vi "autoToteGrab.vi"(8 "potValue":dbl, 9 "# of totes mode":dbl, 10 "ultrasonic":dbl, 11 "Target tracking data":T1) -> (0 "liftMotorOut":dbl, 1 "holonomicRot":dbl, 2 "holonomicY":dbl, 3 "holonomicX":dbl)   [LabVIEW 2014]
uses:
  Robot Global Data.vi
panel:
  in  "totesGrabbed":dbl
  in  "time":dbl
  in  "State":T2(ring)
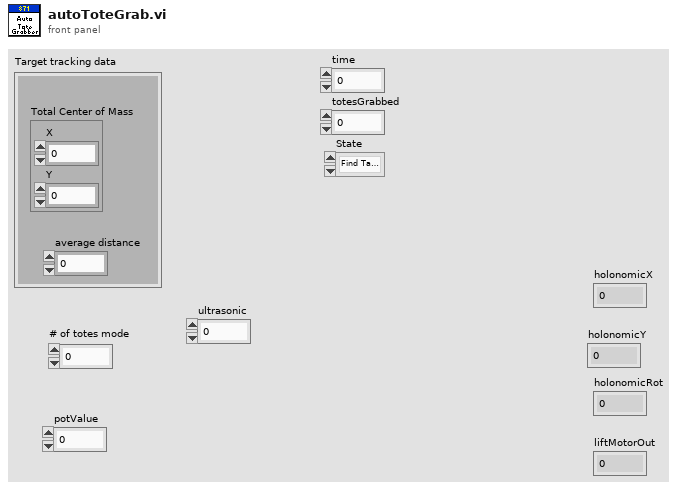
[diagram p1: front panel]
types:
  T1 = cluster{"Total Center of Mass":cluster{"X":dbl, "Y":dbl}, "average distance":dbl}
  T2 = enum16{"Find Targets", "Move to Target", "Prepare to Lift", "Lift Target", "Move Forward", "Drop Totes", "End"}
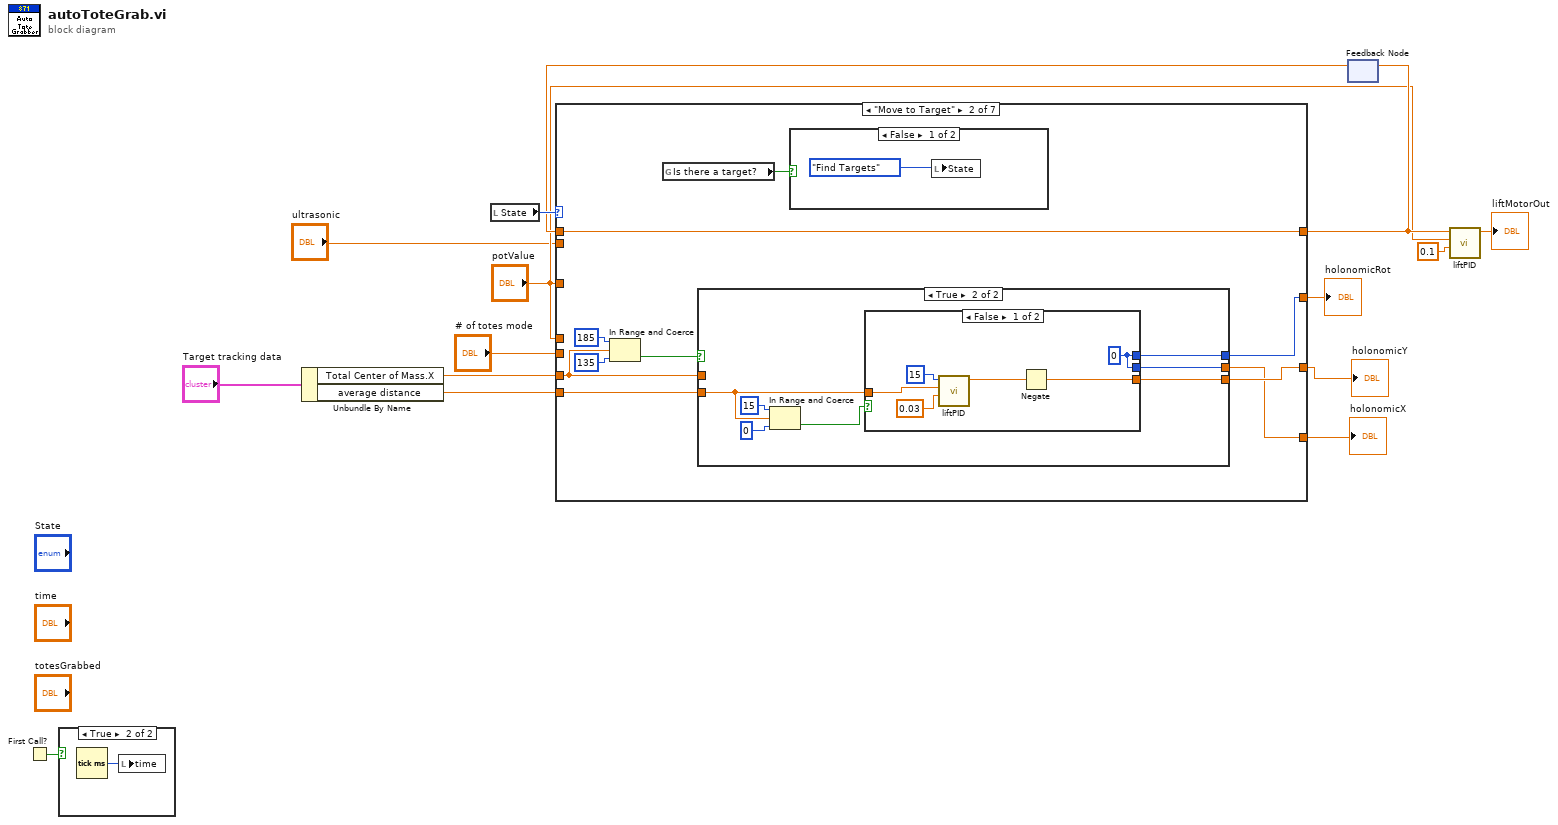
[diagram p0: block diagram]
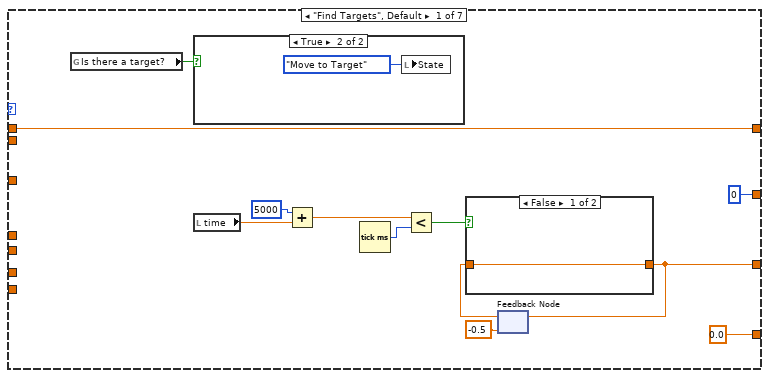
[diagram p3: hidden frame]
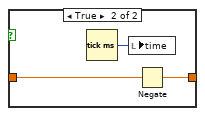
[diagram p4: hidden frame]
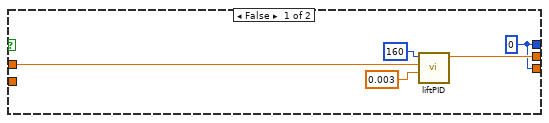
[diagram p7: hidden frame]
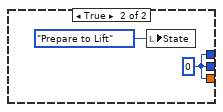
[diagram p8: hidden frame]
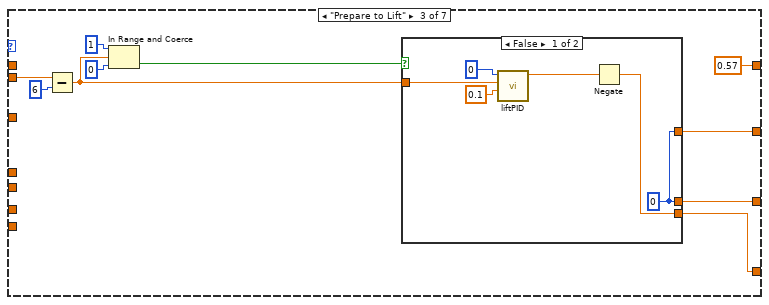
[diagram p9: hidden frame]
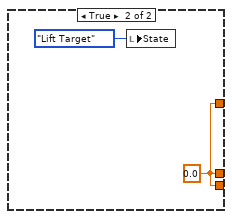
[diagram p10: hidden frame]
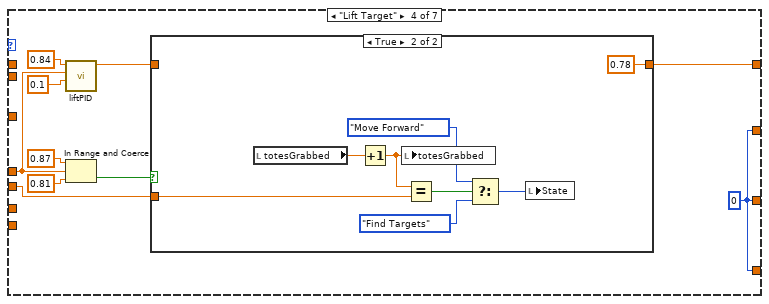
[diagram p11: hidden frame]
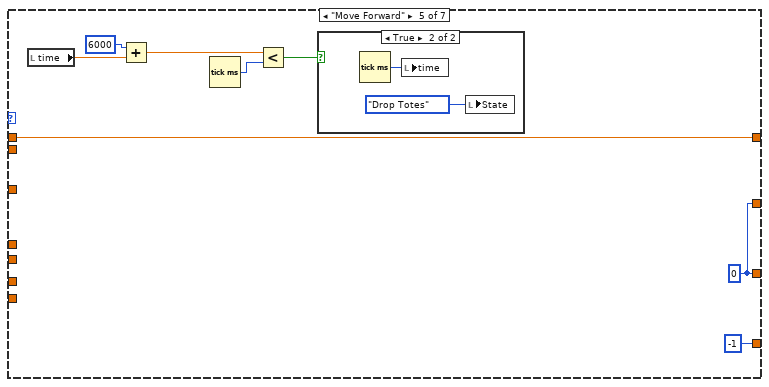
[diagram p13: hidden frame]
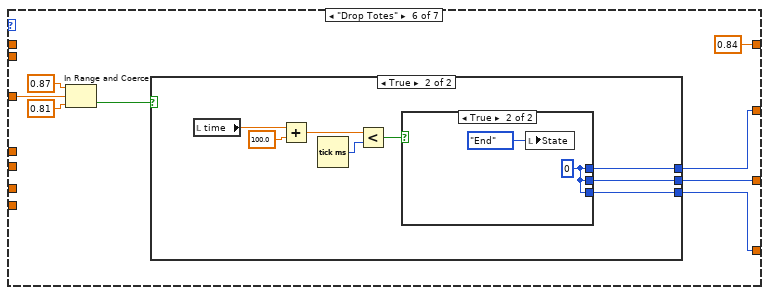
[diagram p15: hidden frame]
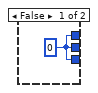
[diagram p16: hidden frame]
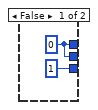
[diagram p17: hidden frame]
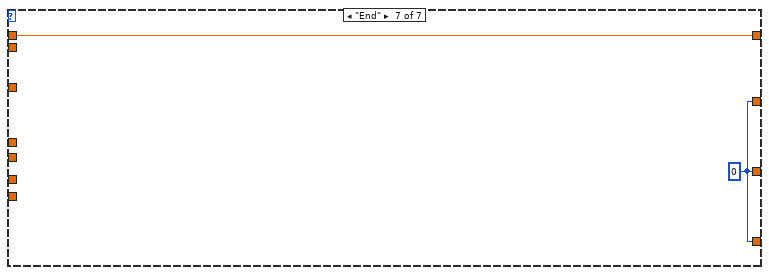
[diagram p18: hidden frame]
diagram:
  n1 = First Call?() -> (First Call?: T/F=w4:bool)
  n2 = case shown="True" w4 {
    frame False {
    }
    frame True {
      n3 = Tick Count (ms)() -> (millisecond timer value=w16:u32)
      n4 = local write "time"(w16) -> ()
    }
  }
  n5 = Unbundle By Name("Target tracking data") -> ("Total Center of Mass.X"=w9:dbl, "average distance"=w8:dbl)
  n6 = local read "State"() -> (w15:T2)
  n7 = feedback #1() -> (w13:dbl)  [unwired: 1 in]
  n8 = case shown="\"Move to Target\"" w15 {
    tunnel: w9 -> [_ w40 _ _ _ _ _]
    tunnel: w8 -> [_ w39 _ _ _ _ _]
    tunnel: "ultrasonic" -> [_ _ w73 _ _ _ _]
    tunnel: "# of totes mode" -> [_ _ _ w92 _ _ _]
    tunnel: [w21 w38 0.57 w85 w104 0.84 w134] -> w12
    tunnel: w13 -> [w21 w38 _ _ w104 _ w134]
    tunnel: "potValue" -> [_ _ _ _ _ w118 _]
    tunnel: [0.0 w34 w66 w84 -1 w113 w133] -> w2
    tunnel: [w19 w35 w67 w84 w102 w114 w133] -> w3
    tunnel: [0 w37 w65 w84 w102 w112 w133] -> w7
    tunnel: "potValue" -> [_ _ _ w83 _ _ _]
    frame "Find Targets", Default {
      n9 = global read "Robot Global Data.vi" "Is there a target?"() -> (w20:bool)
      n10 = case shown="True" w20 {
        frame False {
        }
        frame True {
          n11 = local write "State"(T2."Move to Target" ("State")) -> ()
        }
      }
      n12 = local read "time"() -> (w26:dbl)
      n13 = Add(x=5000, y=w26) -> (x+y=w27:dbl)
      n14 = Tick Count (ms)() -> (millisecond timer value=w28:u32)
      n15 = Less?(x=w27, y=w28) -> (x < y?=w24:bool)
      n16 = feedback #2(-0.5) -> (w23:dbl)
      n17 = case shown="False" w24 {
        tunnel: [w29 w31] -> w19
        tunnel: w23 -> [w29 w30]
        frame False {
        }
        frame True {
          n18 = Tick Count (ms)() -> (millisecond timer value=w32:u32)
          n19 = local write "time"(w32) -> ()
          n20 = Negate(x=w30) -> (-x=w31:dbl)
        }
      }
      n21 = feedback-in #2(w19) -> ()
    }
    frame "Move to Target" {
      n22 = In Range and Coerce(upper limit=185, x=w40, lower limit=135) -> (In Range?=w43:bool)  [unwired: 1 out]
      n23 = global read "Robot Global Data.vi" "Is there a target?"() -> (w36:bool)
      n24 = case shown="True" w43 {
        tunnel: w40 -> [w48 _]
        tunnel: w39 -> [_ w53]
        tunnel: [w46 w52] -> w34
        tunnel: [w45 w51] -> w35
        tunnel: [w45 w50] -> w37
        frame False {
          w45 = 0
          n25 = call "liftPID.vi"("constantProportion"=0.003, "currentValue"=w48, "setValue"=160) -> ("motorOutput"=w46:dbl)  [unwired: 8 in]
        }
        frame True {
          n26 = In Range and Coerce(upper limit=15, x=w53, lower limit=0) -> (In Range?=w56:bool)  [unwired: 1 out]
          n27 = case shown="False" w56 {
            tunnel: w53 -> [w62 _]
            tunnel: [w57 w63] -> w52
            tunnel: [w58 w63] -> w51
            tunnel: [w57 w63] -> w50
            frame False {
              w57 = 0
              n28 = call "liftPID.vi"("constantProportion"=0.03, "currentValue"=w62, "setValue"=15) -> ("motorOutput"=w59:dbl)  [unwired: 8 in]
              n29 = Negate(x=w59) -> (-x=w58:dbl)
            }
            frame True {
              w63 = 0
              n30 = local write "State"(T2."Prepare to Lift" ("State")) -> ()
            }
          }
        }
      }
      n31 = case shown="False" w36 {
        frame False {
          n32 = local write "State"(T2."Find Targets" ("State")) -> ()
        }
        frame True {
        }
      }
    }
    frame "Prepare to Lift" {
      n33 = Subtract(x=w73, y=6) -> (x-y=w69:dbl)
      n34 = In Range and Coerce(upper limit=1, x=w69, lower limit=0) -> (In Range?=w70:bool)  [unwired: 1 out]
      n35 = case shown="False" w70 {
        tunnel: w69 -> [w79 _]
        tunnel: [w75 w81] -> w67
        tunnel: [w76 w81] -> w66
        tunnel: [w75 w81] -> w65
        frame False {
          w75 = 0
          n36 = call "liftPID.vi"("constantProportion"=0.1, "currentValue"=w79, "setValue"=0) -> ("motorOutput"=w77:dbl)  [unwired: 8 in]
          n37 = Negate(x=w77) -> (-x=w76:dbl)
        }
        frame True {
          w81 = 0.0
          n38 = local write "State"(T2."Lift Target" ("State")) -> ()
        }
      }
    }
    frame "Lift Target" {
      w84 = 0
      n39 = call "liftPID.vi"("constantProportion"=0.1, "currentValue"=w83, "setValue"=0.84) -> ("motorOutput"=w89:dbl)  [unwired: 8 in]
      n40 = In Range and Coerce(upper limit=0.87, x=w83, lower limit=0.81) -> (In Range?=w88:bool)  [unwired: 1 out]
      n41 = case shown="True" w88 {
        tunnel: w92 -> [_ w96]
        tunnel: w89 -> [w93 _]
        tunnel: [w93 0.78] -> w85
        frame False {
        }
        frame True {
          n42 = local read "totesGrabbed"() -> (w101:dbl)
          n43 = Increment(x=w101) -> (x+1=w97:dbl)
          n44 = local write "totesGrabbed"(w97) -> ()
          n45 = Equal?(x=w97, y=w96) -> (x = y?=w99:bool)
          n46 = Select(t=T2."Move Forward" ("State"), s=w99, f=T2."Find Targets" ("State")) -> (s? t:f=w98:T2)
          n47 = local write "State"(w98) -> ()
        }
      }
    }
    frame "Move Forward" {
      w102 = 0
      n48 = local read "time"() -> (w109:dbl)
      n49 = Add(x=6000, y=w109) -> (x+y=w107:dbl)
      n50 = Tick Count (ms)() -> (millisecond timer value=w106:u32)
      n51 = Less?(x=w107, y=w106) -> (x < y?=w105:bool)
      n52 = case shown="True" w105 {
        frame False {
        }
        frame True {
          n53 = Tick Count (ms)() -> (millisecond timer value=w110:u32)
          n54 = local write "time"(w110) -> ()
          n55 = local write "State"(T2."Drop Totes" ("State")) -> ()
        }
      }
    }
    frame "Drop Totes" {
      n56 = In Range and Coerce(upper limit=0.87, x=w118, lower limit=0.81) -> (In Range?=w115:bool)  [unwired: 1 out]
      n57 = case shown="True" w115 {
        tunnel: [w120 w122] -> w114
        tunnel: [w120 w123] -> w113
        tunnel: [w120 w121] -> w112
        frame False {
          w120 = 0
        }
        frame True {
          n58 = local read "time"() -> (w128:dbl)
          n59 = Add(x=w128, y=100.0) -> (x+y=w125:dbl)
          n60 = Tick Count (ms)() -> (millisecond timer value=w126:u32)
          n61 = Less?(x=w125, y=w126) -> (x < y?=w124:bool)
          n62 = case shown="True" w124 {
            tunnel: [1 w131] -> w123
            tunnel: [w129 w131] -> w122
            tunnel: [w129 w131] -> w121
            frame False {
              w129 = 0
            }
            frame True {
              w131 = 0
              n63 = local write "State"(T2."End" ("State")) -> ()
            }
          }
        }
      }
    }
    frame "End" {
      w133 = 0
    }
  }
  "holonomicX" <- w2
  "holonomicY" <- w3
  "holonomicRot" <- w7
  n64 = feedback-in #1(w12) -> ()
  n65 = call "liftPID.vi"("constantProportion"=0.1, "currentValue"="potValue", "setValue"=w12) -> ("motorOutput"=→"liftMotorOut":dbl)  [unwired: 8 in]
